vi "Evaluate Part 2.vi"() -> ()   [LabVIEW 2020]
uses:
  Map/Maze.lvclass
panel:
  out "Area":u64
  out "Map out":refnum<class "Maze.lvclass">
  in  "Input":string=".....\n.S-7.\n.|.|.\n.L-J.\n....."
  # "507 too low"
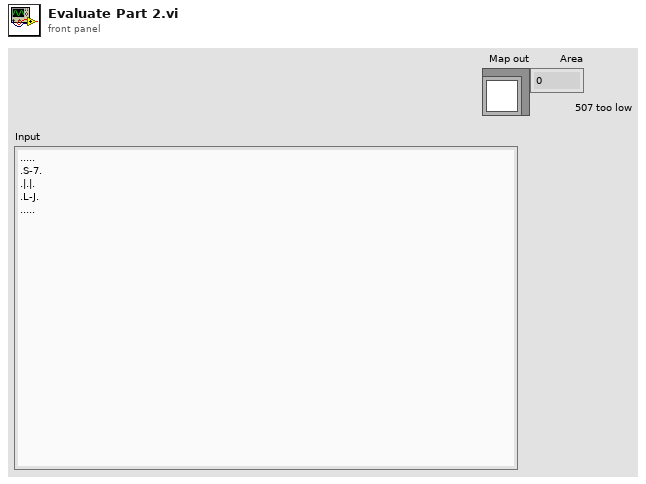
[diagram p1: front panel]
types:
  T1 = typedef "Maze.lvclass/Position.ctl" = cluster{"Row":u64, "Col":u64, "Next Move":enum16{"North", "East", "South", "West", "Halt"}}
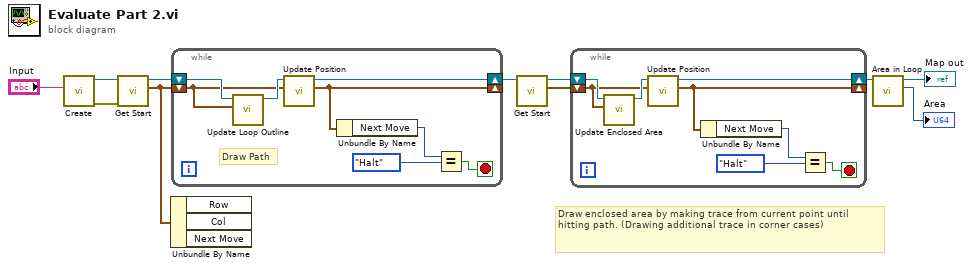
[diagram p0: block diagram]
diagram:
  # "Draw enclosed area by making trace from current point until hitting path. (Drawing additional trace in corner cases)"
  n1 = call "Create.vi"("Input"="Input") -> ("error out"=w10:errorcluster, "Map"=w11:refnum<class "Maze.lvclass">)  [unwired: 9 in]
  n2 = call "Get Start.vi"("error in (no error)"=w10, "Map in"=w11) -> ("Start Vectors"=w1:T1, "Map out"=w2:refnum<class "Maze.lvclass">)  [unwired: 7 in, 1 out]
  n3 = Unbundle By Name(w1) -> ()  [unwired: 3 out]
  n4 = while {
    shift-right: [w18] -> _
    shift-left: w1 -> [w12]
    shift-right: [w15] -> w5
    shift-left: w2 -> [w14]
    stop <- w16 stop-if-true
    # "Draw Path"
    n5 = call "Update Loop Outline.vi"("Start Vectors"=w12, "Map in"=w14) -> ("Map out"=w13:refnum<class "Maze.lvclass">)  [unwired: 9 in]
    n6 = call "Update Position.vi"("Current"=w12, "Map In"=w13) -> ("Next"=w18:T1, "Map Out"=w15:refnum<class "Maze.lvclass">)  [unwired: 6 in, 2 out]
    n7 = Unbundle By Name(w18) -> ("Next Move"=w17:enum16{"North", "East", "South", "West", "Halt"})
    n8 = Equal?(x=w17, y=enum16{"North", "East", "South", "West", "Halt"}."Halt") -> (x = y?=w16:bool)
  }
  n9 = call "Get Start.vi"("Map in"=w5) -> ("Start Vectors"=w4:T1, "Map out"=w3:refnum<class "Maze.lvclass">)  [unwired: 8 in, 1 out]
  n10 = while {
    shift-right: [w26] -> _
    shift-left: w4 -> [w21]
    shift-right: [w20] -> w8
    shift-left: w3 -> [w23]
    stop <- w24 stop-if-true
    n11 = call "Update Enclosed Area.vi"("Start Vectors"=w21, "Map in"=w23) -> ("Map out"=w22:refnum<class "Maze.lvclass">)  [unwired: 9 in]
    n12 = call "Update Position.vi"("Current"=w21, "Map In"=w22) -> ("Next"=w26:T1, "Map Out"=w20:refnum<class "Maze.lvclass">)  [unwired: 6 in, 2 out]
    n13 = Unbundle By Name(w26) -> ("Next Move"=w25:enum16{"North", "East", "South", "West", "Halt"})
    n14 = Equal?(x=w25, y=enum16{"North", "East", "South", "West", "Halt"}."Halt") -> (x = y?=w24:bool)
  }
  n15 = call "Area in Loop.vi"("Map in"=w8) -> ("Area"=→"Area":u64, "Map out"=→"Map out":refnum<class "Maze.lvclass">)  [unwired: 8 in, 1 out]
